vi "Calculate Cascade Feedforward.vi"(11 "Setpoint":dbl) -> (3 "Arbitrary Feedforward":dbl)   [LabVIEW 2020]
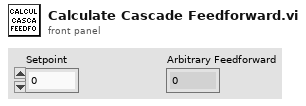
[diagram p1: front panel]
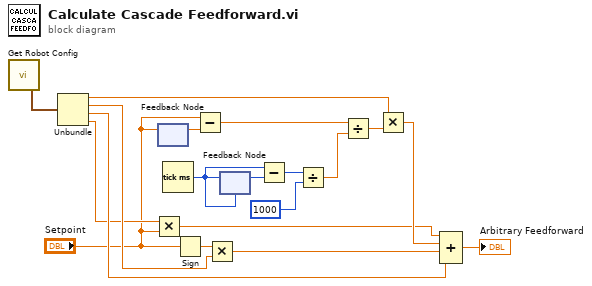
[diagram p0: block diagram]
diagram:
  n1 = call "Get Robot Config.vi"() -> ("Cascade FeedForward Constants"=w4:cluster{"kA":dbl, "kS":dbl, "kG":dbl, "kV":dbl})  [unwired: 12 in, 7 out]
  n2 = Unbundle(w4) -> ("kA"=w7:dbl, "kS"=w6:dbl, "kG"=w5:dbl, "kV"=w3:dbl)
  n3 = Multiply(x=w3, y="Setpoint") -> (x*y=w1:dbl)
  n4 = feedback-in #1("Setpoint") -> ()
  n5 = feedback #1() -> (w17:dbl)  [unwired: 1 in]
  n6 = Tick Count (ms)() -> (millisecond timer value=w14:u32)
  n7 = Sign(1:"Setpoint") -> (0:w19:dbl)
  n8 = Subtract(x="Setpoint", y=w17) -> (x-y=w16:dbl)
  n9 = Multiply(x=w19, y=w6) -> (x*y=w18:dbl)
  n10 = feedback-in #2(w14) -> ()
  n11 = feedback #2(w14) -> (w15:u32)
  n12 = Subtract(x=w14, y=w15) -> (x-y=w13:u32)
  n13 = Divide(x=w13, y=u32 1000) -> (x/y=w11:dbl)
  n14 = Divide(x=w16, y=w11) -> (x/y=w10:dbl)
  n15 = Multiply(x=w7, y=w10) -> (x*y=w9:dbl)
  n16 = Compound Arithmetic op=ADD(w1, w9, w18, w5) -> (→"Arbitrary Feedforward":dbl)
